vi "increament.vi"() -> ()   [LabVIEW 2023]
panel:
  out "Boolean":bool
  in  "OK Button 3":bool
  out "x < y?":bool
  out "x > y?":bool
  out "Numeric":dbl
  in  "UP":bool
  in  "DOWN":bool
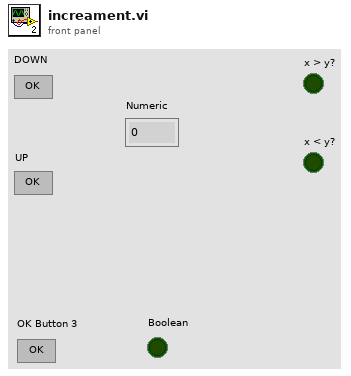
[diagram p1: front panel]
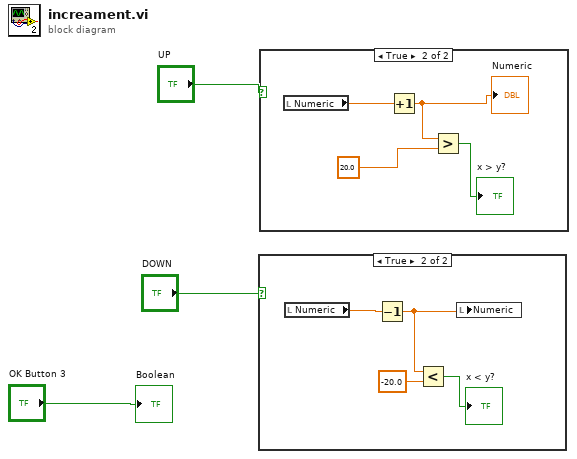
[diagram p0: block diagram]
diagram:
  n1 = case shown="True" "DOWN" {
    frame False {
    }
    frame True {
      n2 = local read "Numeric"() -> (w7:dbl)
      n3 = Decrement(x=w7) -> (x-1=w6:dbl)
      n4 = Less?(x=w6, y=-20.0) -> (x < y?=→"x < y?":bool)
      n5 = local write "Numeric"(w6) -> ()
    }
  }
  n6 = case shown="True" "UP" {
    frame False {
    }
    frame True {
      n7 = local read "Numeric"() -> (w11:dbl)
      n8 = Increment(x=w11) -> (x+1=w10:dbl)
      "Numeric" <- w10
      n9 = Greater?(x=w10, y=20.0) -> (0:→"x > y?":bool)
    }
  }
  "Boolean" <- "OK Button 3"
